vi "Clamp.vi"(8 "error in (no error)":errorcluster, 11 "Instrument.1820 in":refnum<class "Instrument.OxfordVRM.lvclass">) -> (0 "error out":errorcluster, 2 "Response":string, 3 "Instrument.1820 in":refnum<class "Instrument.OxfordVRM.lvclass">)   [LabVIEW 2016, in "Instrument.OxfordVRM.lvclass"]
uses:
  Instrument.OxfordVRM.lvclass
  Typedefs/Instrument.Oxford1820.Commands-enum.ctl
  <instrlib>/Mercury iXX/Public/Libraries/Magnet/Controls/PSU Actions.ctl
  <instrlib>/Mercury iXX/Public/Libraries/Magnet.lvlib
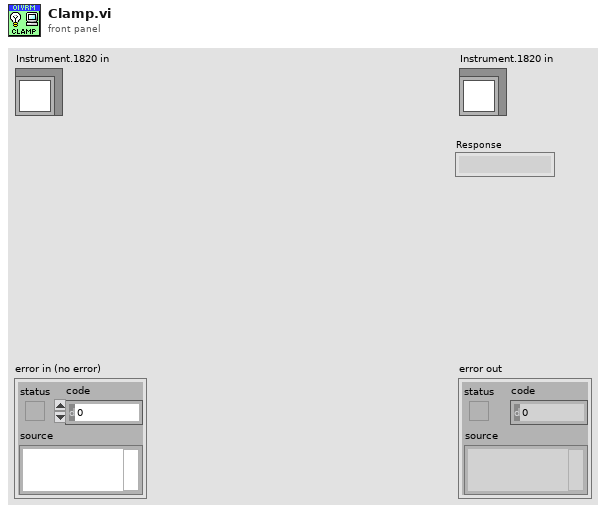
[diagram p1: front panel]
types:
  T1 = typedef "Mercury iXX.lvlib/Magnet.lvlib/PSU Actions.ctl" = string
  T2 = typedef "Instrument.OxfordVRM.lvclass/Instrument.Oxford1820.Commands-enum.ctl" = enum16{"setAction", "setTarget", "setSwitchHeat", "setLambda", "setFillMode", "setNeedleValve", "setMagnetField", "getStatus", "getTarget", "getSwitchHeat", "getPSUField", "newcommand", "getMagnetField"}
  T3 = cluster{"Holding":bool, "Ramp to Setpoint":bool, "Ramp to Zero":bool, "Clamp":bool}
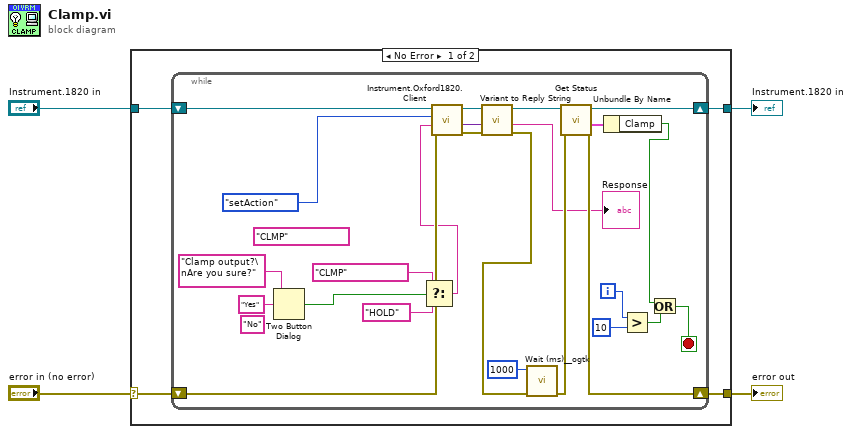
[diagram p0: block diagram]
diagram:
  n1 = case shown="No Error" "error in (no error)" {
    selector: "error in (no error)" -> [w7 w35]
    tunnel: [w5 w35] -> w3
    tunnel: [w6 w34] -> w1
    tunnel: "Instrument.1820 in" -> [w8 w34]
    frame No Error {
      n2 = while {
        shift-right: [w29] -> w6
        shift-left: w8 -> [w26]
        shift-right: [w27] -> w5
        shift-left: w7 -> [w32]
        i -> [w15]
        stop <- w16 stop-if-true
        (unwired) "No" ("F button name (\"Cancel\")")
        (unwired) T1 "CLMP" ("PSU Act Stat")
        n3 = Two Button Dialog(message="Clamp output?\nAre you sure?", 2:"Yes" ("T button name (\"OK\")")) -> (T button?=w24:bool)  [unwired: 1 in]
        n4 = Select(t=T1 "CLMP" ("PSU Act Stat"), s=w24, f=T1 "HOLD" ("PSU Act Stat")) -> (s? t:f=w20:T1)
        n5 = call "Instrument.Oxford1820.Client.vi"("error in (no error)"=w32, "Data"=w20, "Commands"=Instrument.Oxford1820.Commands-enum."setAction", "Instrument.1820 in"=w26) -> ("error out"=w11:errorcluster, "Data out"=w10:variant, "Instrument.1820 out"=w13:refnum<class "Instrument.OxfordVRM.lvclass">)  [unwired: 5 in]
        n6 = call "Variant to Reply String.vi"("error in (no error)"=w11, "Data"=w10, "Instrument.1820 in"=w13) -> ("error out"=w9:errorcluster, "Reply"=→"Response":string, "Instrument.1820 out"=w12:refnum<class "Instrument.OxfordVRM.lvclass">)  [unwired: 6 in]
        n7 = call <userlib>:"Wait (ms)__ogtk.vi"("error in (no error)"=w9, "milliseconds to wait"=u32 1000) -> ("error out"=w28:errorcluster)  [unwired: 8 in, 1 out]
        n8 = call "Get Status.vi"("error in (no error)"=w28, "Instrument.1820 in"=w12) -> ("error out"=w27:errorcluster, "Status"=w30:T3, "Instrument.1820 in"=w29:refnum<class "Instrument.OxfordVRM.lvclass">)  [unwired: 6 in, 1 out]
        n9 = Unbundle By Name(w30) -> ("Clamp"=w17:bool)
        n10 = Greater?(x=w15, y=10) -> (0:w18:bool)
        n11 = Or(x=w17, y=w18) -> (x .or. y?=w16:bool)
      }
    }
    frame Error {
    }
  }
  "error out" <- w3
  "Instrument.1820 in" <- w1
